vi "Write Decoration Index.vi"(3 "DecFrame_FP":refnum<class "DecFrame_FP.lvclass">, 4 "Decoration Index":i32) -> (5 "DecFrame_FP Out":refnum<class "DecFrame_FP.lvclass">)   [LabVIEW 2024, in "DecFrame_FP.lvclass"]
uses:
  DecFrame_FP.lvclass
  DecFrame_FP.lvclass/DecFrame_FP.ctl
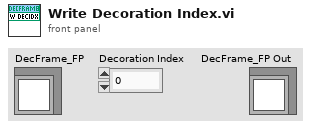
[diagram p1: front panel]
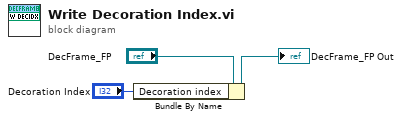
[diagram p0: block diagram]
diagram:
  n1 = Bundle By Name(cluster="DecFrame_FP", "Decoration index"="Decoration Index") -> (→"DecFrame_FP Out":refnum<class "DecFrame_FP.lvclass">)
